vi "isTcpClientQueueFull.vi"(8 "error in (no error)":errorcluster, 11 "tcpServer in":refnum<class "TcpServer.lvclass">) -> (0 "error out":errorcluster, 2 "isTcpClientQueueFull":bool, 3 "tcpServer out":refnum<class "TcpServer.lvclass">)   [LabVIEW 2018, in "TcpServer.lvclass"]
doc: "Check if tcpClientQueue is full to send telemetry to client from component .This returns TRUE if queue is full and FALSE if is not."
uses:
  TcpServer.lvclass
  TcpServer.lvclass/TcpServer.ctl
  TcpServerTel/TcpServerTel.lvclass
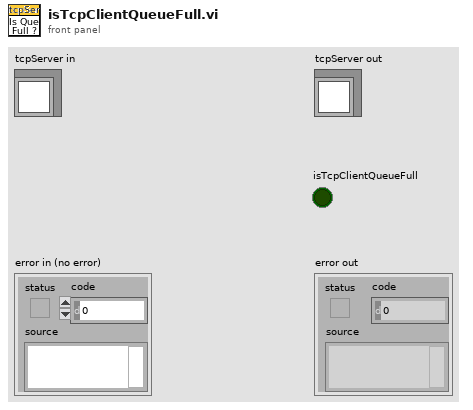
[diagram p1: front panel]
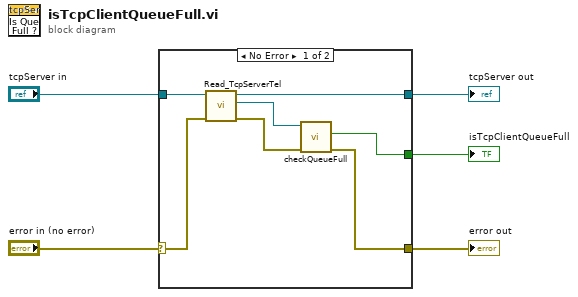
[diagram p0: block diagram]
diagram:
  n1 = case shown="No Error" "error in (no error)" {
    selector: "error in (no error)" -> [w11 w14]
    tunnel: [w8 w14] -> w4
    tunnel: "tcpServer in" -> [w12 w13]
    tunnel: [w7 w13] -> w2
    tunnel: [w6 _] -> w1
    frame No Error {
      n2 = call "Read_TcpServerTel.vi"("error in (no error)"=w11, "TcpServer in"=w12) -> ("error out"=w9:errorcluster, "TcpServerTel.lvclass"=w10:refnum<class "TcpServerTel.lvclass">, "TcpServer out"=w7:refnum<class "TcpServer.lvclass">)  [unwired: 7 in]
      n3 = call "checkQueueFull.vi"("error in (no error)"=w9, "tcpServerTel in"=w10) -> ("error out"=w8:errorcluster, "isTcpClientQueueFull"=w6:bool)  [unwired: 7 in, 1 out]
    }
    frame Error {
    }
  }
  "error out" <- w4
  "tcpServer out" <- w2
  "isTcpClientQueueFull" <- w1
